vi "Average Integration Trigger.vi"(5 "Waveforms":waveform(dbl)[](array[waveform]), 9 "Threshold (V ms)":dbl) -> (6 "Satisfied?":bool, 10 "Average Integration Value":dbl)   [LabVIEW 2013]
panel:
  out "error out":errorcluster
  in  "error in (no error)":errorcluster
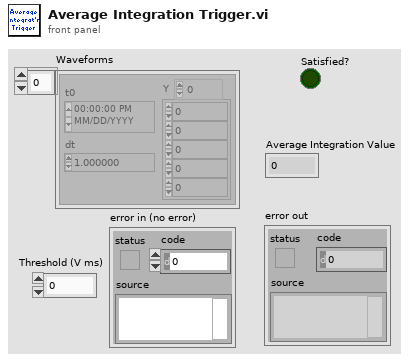
[diagram p1: front panel]
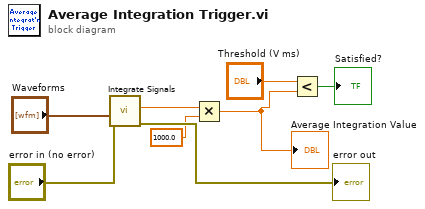
[diagram p0: block diagram]
diagram:
  n1 = call "Integrate Signals.vi"("error in (no error)"="error in (no error)", "Signals"="Waveforms") -> ("error out"=→"error out":errorcluster, "Average Integration Value"=w3:dbl)  [unwired: 6 in, 2 out]
  n2 = Multiply(x=w3, y=1000.0) -> (x*y=w1:dbl)
  "Average Integration Value" <- w1
  n3 = Less?(x="Threshold (V ms)", y=w1) -> (x < y?=→"Satisfied?":bool)
